vi "UTIL_OpenVectorFile.vi"() -> (0 "error out":errorcluster, 1 "Num of Rows":i32, 2 "root path":path, 3 "File Name":string, 4 "Data":dbl[][](array[numeric]), 5 "Cal Coef":dbl[](array[numeric]))   [LabVIEW 2024]
doc: "Opens an Excel file containg Test Vector data defined as follows: \n\nfirst row contains Calibration Coeficients M and B for Level = M * Laser +B \nCol 1 Time in 50 ms\nCol 2 ChA Resistance\nCol 3 ChB Resistance\nCol 4 Laser Output"
uses:
  <vilib>/Utility/NIReport.llb/Excel/NI_Excel.lvclass
  <vilib>/addons/_office/NI_ReportGenerationToolkit.lvlib
  <vilib>/addons/_office/excel.llb/Excel Get Data ([dbl]).vi
  <vilib>/Utility/NIReport.llb/NI_report.lvclass
  <vilib>/Utility/NIReport.llb/Report Type.ctl
  <vilib>/Utility/NIReport.llb/NI_ReportGenerationCore.lvlib
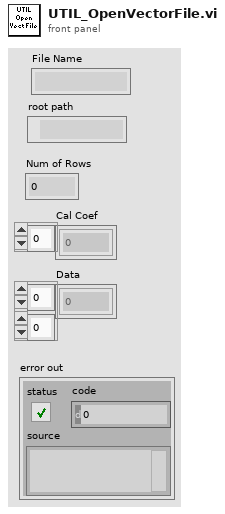
[diagram p1: front panel]
types:
  T1 = typedef "NI_ReportGenerationCore.lvlib/Report Type.ctl" = enum16{"HTML", "Word", "Excel"}
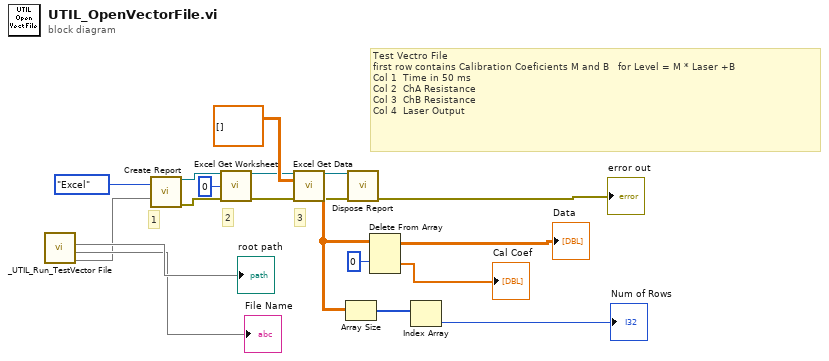
[diagram p0: block diagram]
diagram:
  # "Test Vectro File\nfirst row contains Calibration Coeficients M and B   for Level = M * Laser +B \nCol 1  Time in 50 ms\nCol 2  ChA Resistance\nCol 3  ChB Resistance\nCol 4  Laser Output"
  # "3"
  # "2"
  # "1"
  n1 = call "_UTIL_Run_TestVector File.vi"() -> (0:w1, 1:→"File Name", 2:→"root path")  [unwired: 9 in]
  n2 = call <vilib>:"Create Report.vi"("report type"=Report_Type."Excel", "template (empty)"=w1) -> ("report out"=w9:refnum<class "NI_report.lvclass">, "error out"=w10:errorcluster)  [unwired: 12 in]
  n3 = call <vilib>:"Excel Get Worksheet.vi"("report in"=w9, "worksheet index (0)"=0, "error in (no error)"=w10) -> ("report out"=w7:refnum<class "NI_report.lvclass">, "error out"=w6:errorcluster)  [unwired: 11 in]
  n4 = call-poly <vilib>:"Excel Get Data.vi"("report in"=w7, "data type"=dbl[][] [], "error in (no error)"=w6) -> ("report out"=w18:refnum<class "NI_report.lvclass">, "data"=w15:dbl[][], "error out"=w13:errorcluster)  [unwired: 10 in]
  n5 = Array Size(array=w15) -> (size(s)=w19:i32[])
  n6 = call-dynamic "Dispose Report.vi"("report in"=w18, "error in (no error)"=w13) -> ("error out"=→"error out":errorcluster)  [unwired: 13 in]
  n7 = Delete From Array(array=w15, index (row)=0) -> (deleted portion=→"Cal Coef":dbl[], array with subset deleted=→"Data":dbl[][])  [unwired: 2 in]
  n8 = Index Array(array=w19) -> (element=→"Num of Rows":i32)  [unwired: 1 in]
